vi "Draw Base Minefield.vi"(8 "Error In":errorcluster, 11 "Grid Data":T1[][](array[typedef])) -> (0 "Error Out":errorcluster, 3 "Base Minefield Picture":picture)   [LabVIEW 2011]
doc: "Generates the base image for Minesweeper from an array of mine space information"
uses:
  MineSpace.ctl
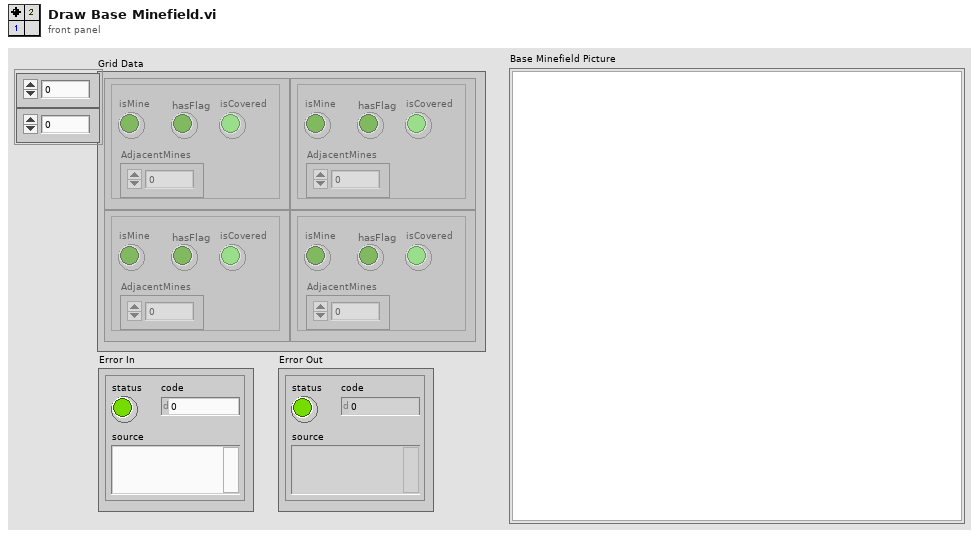
[diagram p1: front panel]
types:
  T1 = typedef "MineSpace.ctl" = cluster{"isMine":bool, "hasFlag":bool, "isCovered":bool, "AdjacentMines":u32}
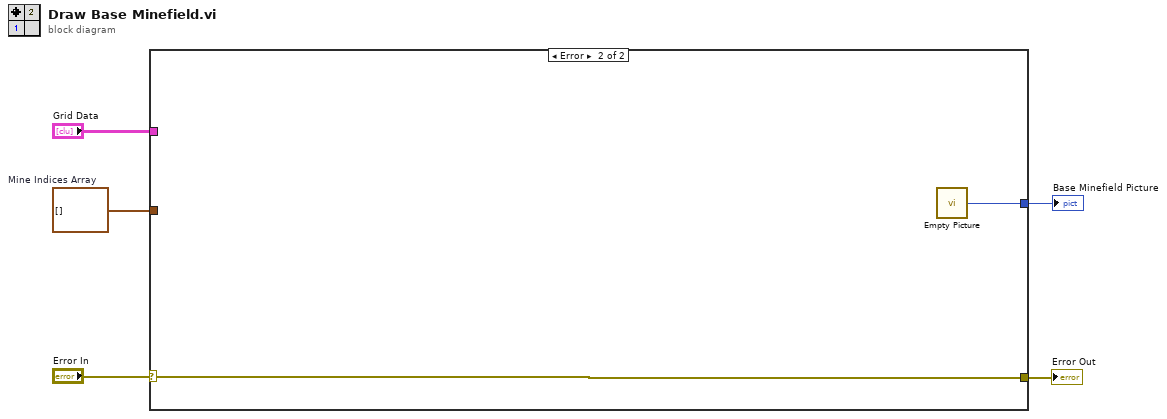
[diagram p0: block diagram]
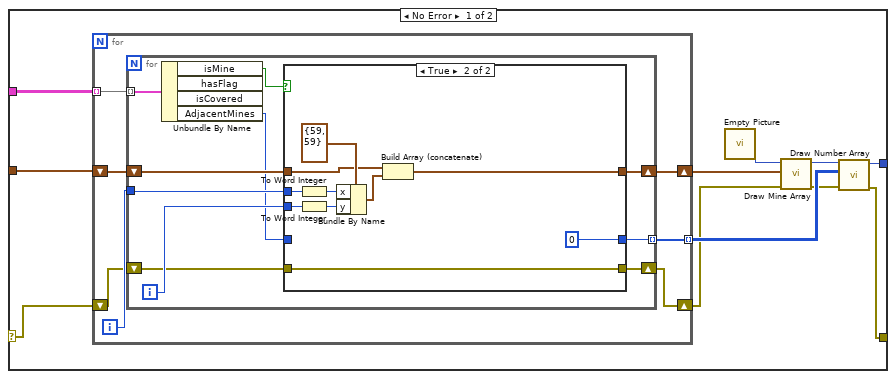
[diagram p2: hidden frame]
diagram:
  w2 = cluster{"x":i16, "y":i16}[] []  # Mine Indices Array
  n1 = case shown="Error" "Error In" {
    selector: "Error In" -> [w6 w48]
    tunnel: "Grid Data" -> [w16 _]
    tunnel: [w11 w47] -> w4
    tunnel: [w8 w48] -> w3
    tunnel: w2 -> [w7 _]
    frame No Error {
      n2 = for {
        tunnel: w16 -> [w23] mode=indexing
        shift-right: [w20] -> w14
        shift-left: w7 -> [w22]
        tunnel: [w19] -> w12 mode=indexing
        shift-right: [w17] -> w10
        shift-left: w6 -> [w18]
        i -> [w21]
        n3 = for {
          tunnel: w23 -> [w33] mode=indexing
          tunnel: w21 -> [w30]
          shift-right: [w28] -> w20
          shift-left: w22 -> [w32]
          tunnel: [w27] -> w19 mode=indexing
          shift-right: [w24] -> w17
          shift-left: w18 -> [w25]
          i -> [w29]
          n4 = Unbundle By Name(w33) -> ("isMine"=w31:bool, "AdjacentMines"=w26:u32)  [unwired: 2 out]
          n5 = case shown="True" w31 {
            tunnel: w32 -> [w36 w41]
            tunnel: w30 -> [_ w44]
            tunnel: w29 -> [_ w42]
            tunnel: [w36 w39] -> w28
            tunnel: [w35 u32 0] -> w27
            tunnel: w26 -> [w35 _]
            tunnel: w25 -> [w34 w37]
            tunnel: [w34 w37] -> w24
            frame False {
            }
            frame True {
              n6 = To Word Integer(number=w44) -> (16bit integer=w45:i16)
              n7 = To Word Integer(number=w42) -> (16bit integer=w43:i16)
              n8 = Bundle By Name(cluster=cluster{"x":i16, "y":i16} {"x"=59, "y"=59} ("new position"), "x"=w45, "y"=w43) -> (w40:cluster{"x":i16, "y":i16})
              n9 = Build Array (concatenate)(w41, w40) -> (w39:cluster{"x":i16, "y":i16}[])
            }
          }
        }
      }
      n10 = call "Empty Picture"() -> ("empty picture"=w15:picture)
      n11 = call "Draw Mine Array.vi"("Error In"=w10, "Box Array"=w14, "Picture In"=w15) -> ("Error Out"=w9:errorcluster, "Picture Out"=w13:picture)  [unwired: 7 in]
      n12 = call "Draw Number Array.vi"("Error In"=w9, "Number of Mines Array"=w12, "Picture In"=w13) -> ("Error Out"=w8:errorcluster, "Picture Out"=w11:picture)  [unwired: 7 in]
    }
    frame Error {
      n13 = call "Empty Picture"() -> ("empty picture"=w47:picture)
    }
  }
  "Base Minefield Picture" <- w4
  "Error Out" <- w3
